vi "getStatesByChannelName.vi"(8 "error in (no error)":errorcluster, 10 "channel_name":string, 11 "ChannelArray in":refnum<class "ChannelArray.lvclass">) -> (0 "error out":errorcluster, 2 "states":cluster{"state_name":string, "value":string}[](array[cluster]), 3 "ChannelArray out":refnum<class "ChannelArray.lvclass">)   [LabVIEW 2009, in "Tools.lvlib" / "DatabaseHelpers.lvlib" / "ChannelArray.lvclass"]
uses:
  ChannelArray.lvclass
  Channel/Channel.lvclass
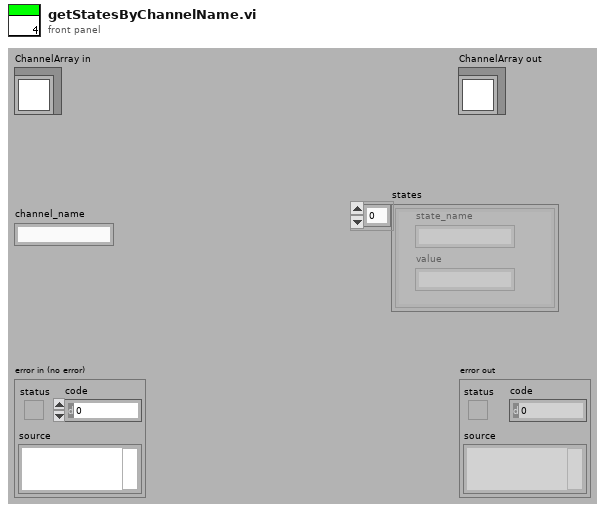
[diagram p1: front panel]
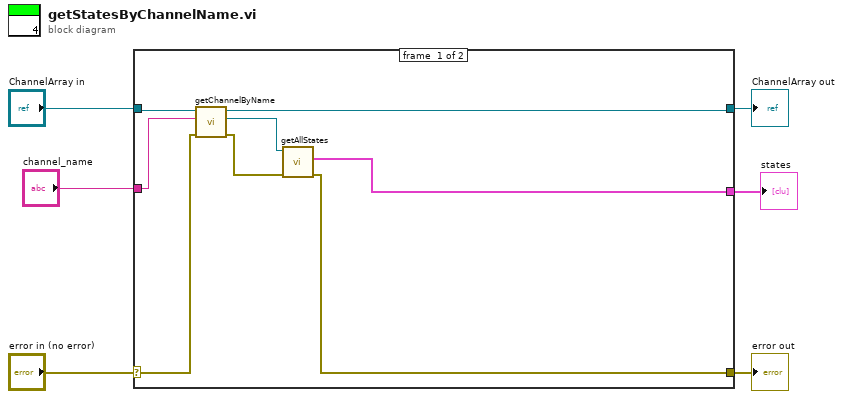
[diagram p0: block diagram]
diagram:
  n1 = case shown="No Error" "error in (no error)" {
    selector: "error in (no error)" -> [w12 w16]
    tunnel: [w7 w16] -> w5
    tunnel: [w11 w15] -> w3
    tunnel: "ChannelArray in" -> [w14 w15]
    tunnel: "channel_name" -> [w13 _]
    tunnel: [w9 _] -> w1
    frame #0 {
      n2 = call-dynamic "getChannelByName.vi"("error in (no error)"=w12, "channel_name"=w13, "ChannelArray in"=w14) -> ("error out"=w8:errorcluster, "Channel"=w10:refnum<class "Channel.lvclass">, "ChannelArray out"=w11:refnum<class "ChannelArray.lvclass">)  [unwired: 5 in, 1 out]
      n3 = call "getAllStates.vi"("error in (no error)"=w8, "Channel.lvclass in"=w10) -> ("error out"=w7:errorcluster, "states"=w9:cluster{"state_name":string, "value":string}[])  [unwired: 7 in, 1 out]
    }
    frame #1 {
    }
  }
  "error out" <- w5
  "ChannelArray out" <- w3
  "states" <- w1
